vi "Save GIF Image (UTF-8 Path).vi"(8 "error in (no error)":errorcluster, 9 "Dither (None)":T1, 10 "Image":T2, 11 "Path In":string) -> (0 "error out":errorcluster, 3 "Path Out":string)   [LabVIEW 2020, in "G-Image.lvlib"]
doc: "Saves an image in GIF format to disk.\n\nTrue color images will be automatically quantized to 8-bit using a median-cut filter, and optional dithering. This process can be slow for large images.\n\n8-bit images are written directly to the GIF file.s"
uses:
  G-Image.lvlib
  <vilib>/picture/picture.llb/imagedata.ctl
  Controls/Dither Type.ctl
  Controls/Image Save Format.ctl
  4e92731f-a350-4349-bfa5-6fae956bbb92.vi
  Private/Result To Error.vi
  Private/Get Image Data.vi
  Private/ARGB To RGBA.vi
  Private/Depth To Number Channels.vi
  Image Processing/Indexed Color To True Color Image.vi
  <vilib>/Utility/error.llb/Error Cluster From Error Code.vi
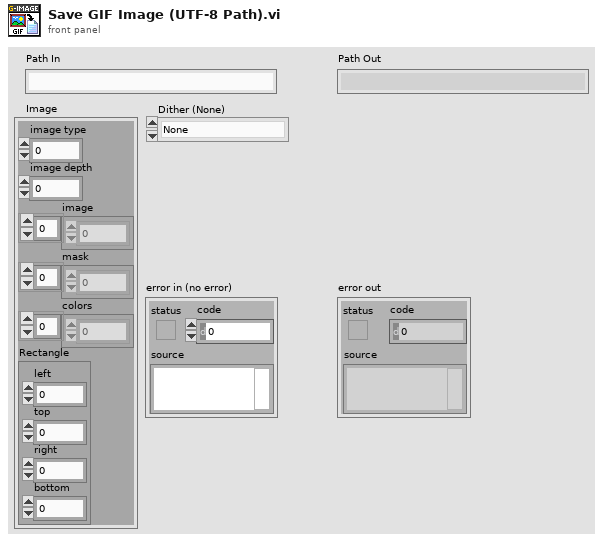
[diagram p1: front panel]
types:
  T1 = typedef "G-Image.lvlib/Dither Type.ctl" = enum32{"None", "Floyd-Steinberg"}
  T2 = typedef "imagedata.ctl" = cluster{"image type":i32, "image depth":i32, "image":u8[], "mask":u8[], "colors":u32[], "Rectangle":cluster{"left":i16, "top":i16, "right":i16, "bottom":i16}}
  T3 = typedef "G-Image.lvlib/Image Save Format.ctl" = enum16{"png", "jpg", "bmp", "gif", "tga"}
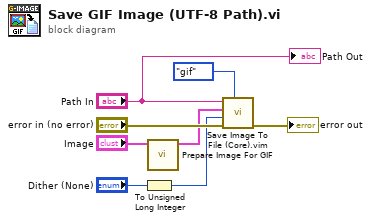
[diagram p0: block diagram]
diagram:
  n1 = To Unsigned Long Integer(number="Dither (None)") -> (unsigned 32bit integer=w2:u32)
  n2 = call "Prepare Image For GIF.vi"("Image"="Image") -> ("Image"=w3:T2)  [unwired: 9 in, 1 out]
  n3 = call "Save Image To File (Core).vim"("Save Format"=Image_Save_Format."gif", "error in (no error)"="error in (no error)", "Option"=w2, "Picture"=w3, "Path In"="Path In") -> ("error out"=→"error out":errorcluster)  [unwired: 5 in, 1 out]
  "Path Out" <- "Path In"
